vi "S2C_UNITHERM_Proc_Custom.vi"(7 "Local?":bool, 8 "Error In":errorcluster, 10 "Command":string, 11 "JSON String":string) -> (0 "Error Out":errorcluster, 3 "Response":variant)   [LabVIEW 2024]
uses:
  S2C_UNITHERM_Proc_Globals.vi
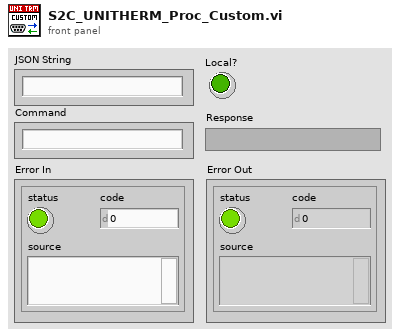
[diagram p1: front panel]
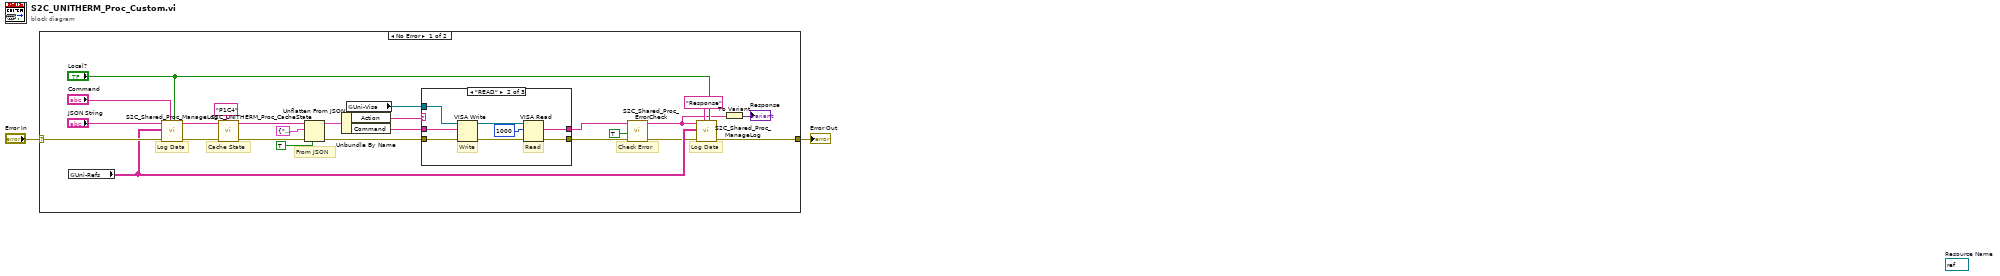
[diagram p0: block diagram]
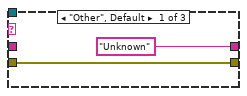
[diagram p2: hidden frame]
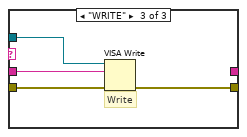
[diagram p3: hidden frame]
diagram:
  (unwired) refnum<visa-resource-name> refnum  # Resource Name
  n1 = case shown="No Error" "Error In" {
    selector: "Error In" -> [w20 w42]
    tunnel: [w17 w42] -> w1
    frame No Error {
      # "Check Error"
      # "Cache State"
      # "Log Data"
      # "Log Data"
      # "From JSON"
      n2 = global read "S2C_UNITHERM_Proc_Globals.vi" "Uni-Refs"() -> (w9:string[][])
      n3 = call "S2C_Shared_Proc_ManageLog.vi"("Local?"="Local?", "Command"="Command", "Error In"=w20, "Refs"=w9, "Data In"="JSON String") -> ("Error Out"=w13:errorcluster, "Data Out"=w11:string)  [unwired: 5 in]
      n4 = call "S2C_UNITHERM_Proc_CacheState.vi"("Label"="P1C4", "Error In"=w13, "Data In"=w11) -> ("Error Out"=w12:errorcluster, "Data Out"=w10:string)  [unwired: 7 in]
      n5 = Unflatten From JSON(JSON string=w10, type and defaults=cluster{"Command":string, "Action":string} {"Command"="", "Action"=""}, default null elements? (F)=TRUE, error in (no error)=w12) -> (value=w26:cluster{"Command":string, "Action":string}, error out=w24:errorcluster)  [unwired: 3 in]
      n6 = Unbundle By Name(w26) -> ("Action"=w21:string, "Command"=w23:string)
      n7 = global read "S2C_UNITHERM_Proc_Globals.vi" "Uni-Visa"() -> (w3:refnum<visa-resource-name>)
      n8 = case shown="\"READ\"" w21 {
        tunnel: [w29 w34 w38] -> w8
        tunnel: w24 -> [w29 w33 w41]
        tunnel: w23 -> [_ w32 w40]
        tunnel: w3 -> [_ w31 w39]
        tunnel: ["Unknown" ("read buffer") w30 _] -> w7
        frame "Other", Default {
        }
        frame "READ" {
          # "Read"
          # "Write"
          n9 = VISA Write(VISA resource name=w31, write buffer=w32, error in (no error)=w33) -> (VISA resource name out=w36:refnum<visa-resource-name>, error out=w37:errorcluster)  [unwired: 1 out]
          n10 = VISA Read(VISA resource name=w36, byte count=u32 1000, error in (no error)=w37) -> (read buffer=w30:string, error out=w34:errorcluster)  [unwired: 2 out]
        }
        frame "WRITE" {
          # "Write"
          n11 = VISA Write(VISA resource name=w39, write buffer=w40, error in (no error)=w41) -> (error out=w38:errorcluster)  [unwired: 2 out]
        }
      }
      n12 = call "S2C_Shared_Proc_ErrorCheck.vi"("Error In"=w8, "ExpReply?"=TRUE, "Reply Text"=w7) -> ("Error Out"=w5:errorcluster, "Status"=w6:string)  [unwired: 7 in]
      n13 = call "S2C_Shared_Proc_ManageLog.vi"("Local?"="Local?", "Command"="Response", "Error In"=w5, "Refs"=w9, "Data In"=w6) -> ("Error Out"=w17:errorcluster)  [unwired: 5 in, 1 out]
      n14 = To Variant(anything=w6) -> (Variant=→"Response":variant)
    }
    frame Error {
    }
  }
  "Error Out" <- w1
